vi "Calc_Scrub_Array.vi"(0 "Start":i32, 4 "Stop":i32, 7 "Array in":dbl[](array[numeric])) -> (23 "Array out":dbl[](array[numeric]))   [LabVIEW 2025]
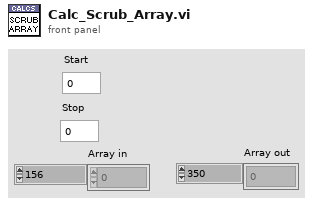
[diagram p1: front panel]
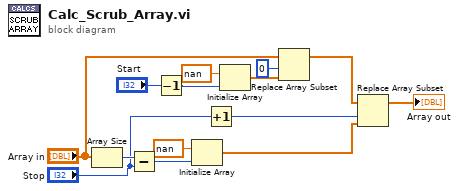
[diagram p0: block diagram]
diagram:
  n1 = Array Size(array="Array in") -> (size(s)=w12:i32)
  n2 = Subtract(x=w12, y="Stop") -> (x-y=w10:i32)
  n3 = Decrement(x="Start") -> (x-1=w7:i32)
  n4 = Initialize Array(nan ("element"), w10) -> (w5:dbl[])
  n5 = Increment(x="Stop") -> (x+1=w3:i32)
  n6 = Initialize Array(nan ("element"), w7) -> (w8:dbl[])
  n7 = Replace Array Subset(array="Array in", new element=w8, index=0) -> (w6:dbl[])
  n8 = Replace Array Subset(array=w6, new element=w5, index=w3) -> (→"Array out":dbl[])
